vi "Finish.vi"   [LabVIEW 2011]
doc: "This VI is called just before exiting. It is expected to close I/O refnum, save collected data, etc."
types:
  T1 = typedef "WPI_DigitalInputDevRef.ctl" = cluster{"DevStatus":errorcluster, "DIO Channel":T2, "Digital Module":T3}
  T2 = typedef "FPGA_DIOChannel.ctl" = enum8{"DIO 1", "DIO 2", "DIO 3", "DIO 4", "DIO 5", "DIO 6", "DIO 7", "DIO 8", "DIO 9", "DIO 10", "DIO 11", "DIO 12", "DIO 13", "DIO 14", "Invalid"}
  T3 = typedef "FPGA_TypedefDigitalModule.ctl" = enum16{"Digital Module 1", "Digital Module 2"}
  T4 = typedef "WPI_CameraDevRef.ctl" = cluster{"Camera Address":string, "CameraStatus":errorcluster, "Acquire Image Notifier":refnum<notifier>}
  T5 = typedef "WPI_JoystickDevRef.ctl" = cluster{"Device":T6}
  T6 = typedef "WPI_JoystickDeviceEnum.ctl" = enum16{"USB 1", "USB 2", "USB 3", "USB 4", "Kinect 1", "Kinect 2"}
  T7 = typedef "WPI_RelayDevRef.ctl" = cluster{"DevStatus":errorcluster, "Relay Channel":T8, "Digital Module":T3, "Relay Direction":T9}
  T8 = typedef "FPGA_DIORelayChannel.ctl" = enum8{"Relay 1", "Relay 2", "Relay 3", "Relay 4", "Relay 5", "Relay 6", "Relay 7", "Relay 8", "Invalid"}
  T9 = typedef "WPI_RelayDirection.ctl" = enum16{"Both directions", "Forward only", "Reverse only"}
  T10 = typedef "WPI_MotorControlDeviceRef.ctl" = cluster{"DeviceStatus":errorcluster, "Type":enum16{"PWM", "CAN"}, "PWM":cluster{"Digital Module":T3, "PWM Channel":T11, "DeadBand":T12}, "CAN":cluster{"Device Number":u8, "Control Mode":T13, "Semaphore":T14, "Max Vout":dbl}, "Invert":bool, "TransformRef":T15, "InvTransformRef":T15}
  T11 = typedef "FPGA_DIOPWMChannel.ctl" = enum8{"PWM 1", "PWM 2", "PWM 3", "PWM 4", "PWM 5", "PWM 6", "PWM 7", "PWM 8", "PWM 9", "PWM 10", "Invalid"}
  T12 = typedef "WPI_PWMDeadband.ctl" = cluster{"Name":string, "maxPositivePwm":i32, "minPositivePwm":i32, "centerPwm":i32, "maxNegativePwm":i32, "minNegativePwm":i32, "angularRange":u16}
  T13 = typedef "WPI_CANJaguar_ControlMode.ctl" = enum8{"Percent VBus", "Current", "Speed", "Position", "Voltage"}
  T14 = typedef "Semaphore RefNum" = refnum<k1>
  T15 = typedef "WPI_PWMTransform_ConPane.ctl" = refnum<vi>
  T16 = typedef "WPI_RobotDriveDevRef.ctl" = cluster{"DevStatus":errorcluster, "Motors[]":T10[], "Square Inputs":bool, "Max Output":dbl, "Isochronous":bool}
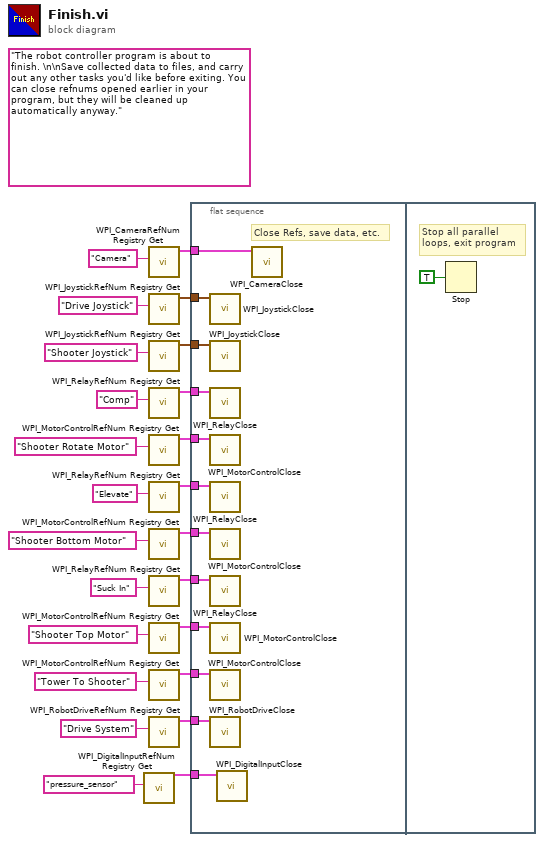
[diagram p0: block diagram]
diagram:
  (unwired) "The robot controller program is about to finish. \n\nSave collected data to files, and carry out any other tasks you'd like before exiting. You can close refnums opened earlier in your program, but they will be cleaned up automatically anyway."
  n1 = call <vilib>:"WPI_DigitalInputRefNum Registry Get.vi"("refnum name"="pressure_sensor") -> ("DigitalInputDevRef"=w2:T1)  [unwired: 9 in, 1 out]
  n2 = call <vilib>:"WPI_CameraRefNum Registry Get.vi"("refnum name"="Camera") -> ("CameraDevRef"=w20:T4)  [unwired: 1 in, 9 out]
  n3 = call <vilib>:"WPI_JoystickRefNum Registry Get.vi"("refnum name"="Drive Joystick") -> ("JoystickDevRef"=w21:T5)  [unwired: 1 in, 9 out]
  n4 = call <vilib>:"WPI_JoystickRefNum Registry Get.vi"("refnum name"="Shooter Joystick") -> ("JoystickDevRef"=w17:T5)  [unwired: 1 in, 9 out]
  n5 = call <vilib>:"WPI_RelayRefNum Registry Get.vi"("refnum name"="Comp") -> ("RelayDevRef"=w4:T7)  [unwired: 9 in, 1 out]
  n6 = call <vilib>:"WPI_MotorControlRefNum Registry Get.vi"("refnum name"="Shooter Rotate Motor") -> ("MotorControlDevRef"=w16:T10)  [unwired: 9 in, 1 out]
  n7 = call <vilib>:"WPI_RelayRefNum Registry Get.vi"("refnum name"="Elevate") -> ("RelayDevRef"=w9:T7)  [unwired: 9 in, 1 out]
  n8 = call <vilib>:"WPI_MotorControlRefNum Registry Get.vi"("refnum name"="Shooter Bottom Motor") -> ("MotorControlDevRef"=w15:T10)  [unwired: 9 in, 1 out]
  n9 = call <vilib>:"WPI_RelayRefNum Registry Get.vi"("refnum name"="Suck In") -> ("RelayDevRef"=w10:T7)  [unwired: 9 in, 1 out]
  n10 = call <vilib>:"WPI_MotorControlRefNum Registry Get.vi"("refnum name"="Shooter Top Motor") -> ("MotorControlDevRef"=w14:T10)  [unwired: 9 in, 1 out]
  n11 = call <vilib>:"WPI_MotorControlRefNum Registry Get.vi"("refnum name"="Tower To Shooter") -> ("MotorControlDevRef"=w6:T10)  [unwired: 9 in, 1 out]
  n12 = call <vilib>:"WPI_RobotDriveRefNum Registry Get.vi"("refnum name"="Drive System") -> ("RobotDriveDevRef"=w22:T16)  [unwired: 1 in, 9 out]
  n13 = flat-sequence {
    tunnel: w22 -> [w36]
    tunnel: w21 -> [w35]
    tunnel: w20 -> [w34]
    tunnel: w17 -> [w33]
    tunnel: w16 -> [w32]
    tunnel: w15 -> [w31]
    tunnel: w14 -> [w30]
    tunnel: w10 -> [w29]
    tunnel: w9 -> [w28]
    tunnel: w6 -> [w27]
    tunnel: w4 -> [w26]
    tunnel: w2 -> [w25]
    frame #0 {
      # "Close Refs, save data, etc."
      n14 = call <vilib>:"WPI_JoystickClose.vi"("JoystickDevRef"=w35) -> ()  [unwired: 11 out]
      n15 = call <vilib>:"WPI_JoystickClose.vi"("JoystickDevRef"=w33) -> ()  [unwired: 11 out]
      n16 = call <vilib>:"WPI_RelayClose.vi"("RelayDevRef"=w26) -> ()  [unwired: 10 in, 1 out]
      n17 = call <vilib>:"WPI_MotorControlClose.vi"("MotorControlDevRef"=w32) -> ()  [unwired: 10 in, 1 out]
      n18 = call <vilib>:"WPI_RelayClose.vi"("RelayDevRef"=w28) -> ()  [unwired: 10 in, 1 out]
      n19 = call <vilib>:"WPI_MotorControlClose.vi"("MotorControlDevRef"=w31) -> ()  [unwired: 10 in, 1 out]
      n20 = call <vilib>:"WPI_RelayClose.vi"("RelayDevRef"=w29) -> ()  [unwired: 10 in, 1 out]
      n21 = call <vilib>:"WPI_MotorControlClose.vi"("MotorControlDevRef"=w30) -> ()  [unwired: 10 in, 1 out]
      n22 = call <vilib>:"WPI_MotorControlClose.vi"("MotorControlDevRef"=w27) -> ()  [unwired: 10 in, 1 out]
      n23 = call <vilib>:"WPI_RobotDriveClose.vi"("RobotDriveDevRef"=w36) -> ()  [unwired: 1 in, 10 out]
      n24 = call <vilib>:"WPI_DigitalInputClose.vi"("DigitalInputDevRef"=w25) -> ()  [unwired: 10 in, 1 out]
      n25 = call <vilib>:"WPI_CameraClose.vi"("CameraDevRef"=w34) -> ()  [unwired: 1 in, 10 out]
    }
    frame #1 {
      # "Stop all parallel\nloops, exit program"
      n26 = Stop(stop? (T)=TRUE ("Quit")) -> ()
    }
  }
